vi "FTW-Message-Request-Reply.vi"(8 "error in":errorcluster, 9 "Response Body":string, 10 "Response Header":string, 11 "FTW Incoming Request":refnum<class "FTW-Message-IncomingRequest.lvclass">) -> (0 "error out":errorcluster, 2 "Timed out?":bool)   [LabVIEW 2012, in "FTW-Actor.lvlib" / "FTW-Message-IncomingRequest.lvclass"]
uses:
  FTW-Message-IncomingRequest.lvclass
  FTW-Message-IncomingRequest.lvclass/FTW-Message-IncomingRequest.ctl
  Endpoint/FTW-Endpoint.lvclass
panel:
  # "Inputs"
  # "Outputs"
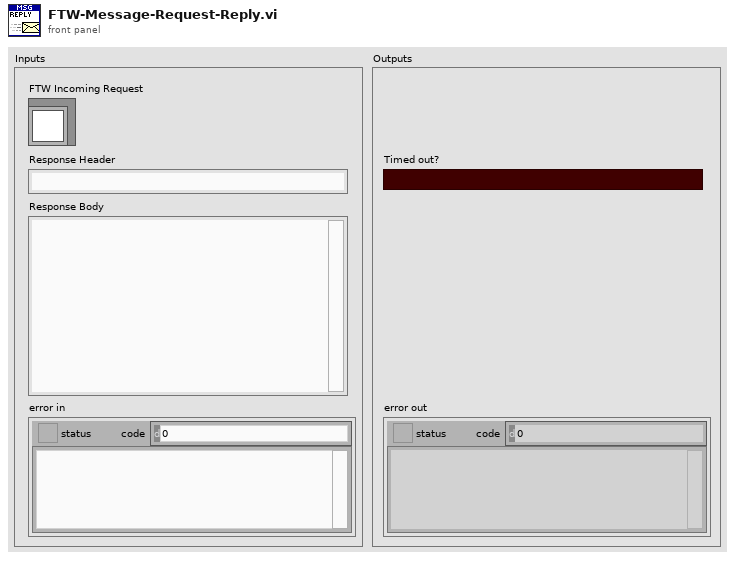
[diagram p1: front panel]
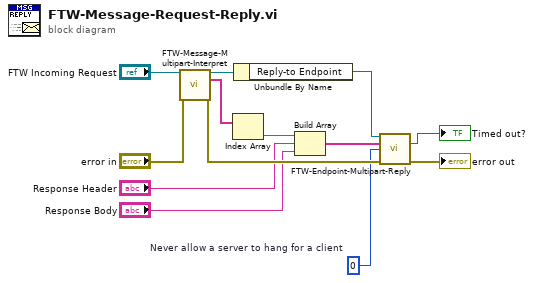
[diagram p0: block diagram]
diagram:
  w2 = 0  # Never allow a server to hang for a client
  n1 = call-dynamic "FTW-Message-Multipart-Interpret.vi"("FTW Message"="FTW Incoming Request", "error in"="error in") -> ("FTW Message out"=w11:refnum<class "FTW-Message-IncomingRequest.lvclass">, "Message Parts"=w9:string[], "error out"=w13:errorcluster)  [unwired: 11 in]
  n2 = Index Array(array=w9) -> (element=w7:string)  [unwired: 1 in]
  n3 = Unbundle By Name(w11) -> ("Reply-to Endpoint"=w6:refnum<class "FTW-Endpoint.lvclass">)
  n4 = Build Array(w7, "Response Header", "Response Body") -> (w8:string[])
  n5 = call-dynamic "FTW-Endpoint-Multipart-Reply.vi"("FTW Endpoint"=w6, "Multipart Message"=w8, "Timeout"=w2, "error in"=w13) -> ("Timed out?"=→"Timed out?":bool, "error out"=→"error out":errorcluster)  [unwired: 9 in, 1 out]
